vi "SubVI_SA_ReadMarker.vi"(8 "error in (no error)":errorcluster, 10 "AvgTimes":i32=1, 11 "VISA resource name":refnum<visa-resource-name>="TCPIP0::192.168.100.230::inst0::INSTR") -> (0 "error out":errorcluster, 1 "Marker Freq.":dbl, 3 "VISA resource name out":refnum<visa-resource-name>, 4 "Marker Power":dbl format="%.3f")   [LabVIEW 2023]
uses:
  Anritsu Signal Analyzer Series/Public/Data/Read Marker (Active Marker).vi
  Anritsu Signal Analyzer Series/Anritsu Signal Analyzer Series.lvlib
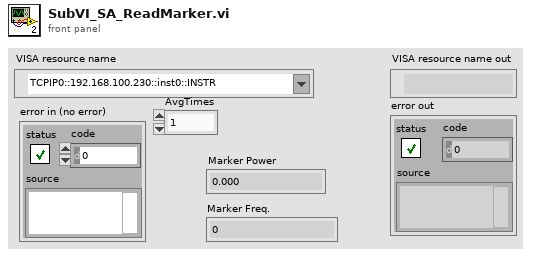
[diagram p1: front panel]
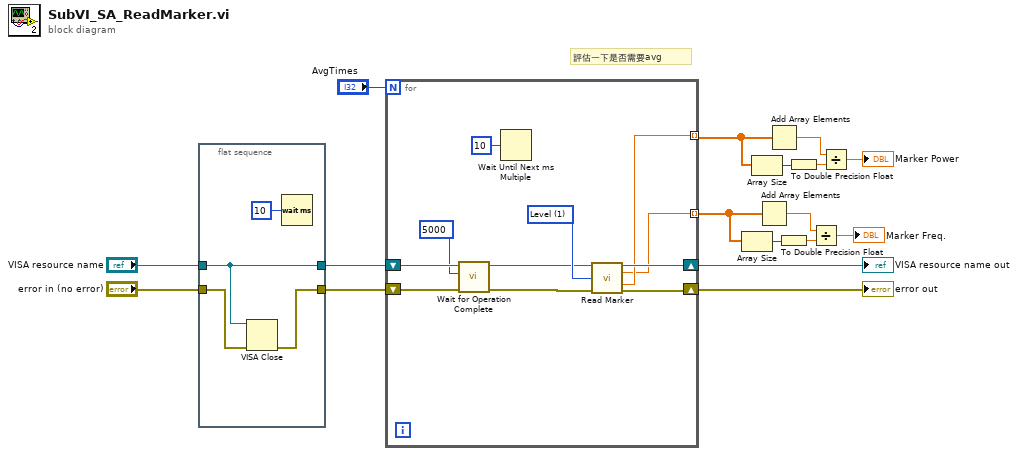
[diagram p0: block diagram]
diagram:
  # "評估一下是否需要avg"
  n1 = flat-sequence {
    tunnel: "error in (no error)" -> [w20]
    tunnel: [w19] -> w9
    tunnel: "VISA resource name" -> [w18]
    tunnel: [w18] -> w7
    frame #0 {
      n2 = VISA Close(VISA resource name=w18, error in (no error)=w20) -> (error out=w19:errorcluster)
      n3 = Wait (ms)(milliseconds to wait=u32 10) -> ()  [unwired: 1 out]
    }
  }
  n4 = for {
    N: "AvgTimes" -> [_]
    shift-right: [w27] -> w17
    shift-left: w7 -> [w29]
    shift-right: [w26] -> w16
    shift-left: w9 -> [w28]
    tunnel: [w25] -> w15 mode=indexing
    tunnel: [w23] -> w1 mode=indexing
    w32 = 1 items=["Frequency or Time", "Level", "Position"] ("Marker Type (0:Frequency or Time)")
    n5 = call "Wait for Operation Complete.vi"("error in (no error)"=w28, "Maximum Time (10000mSec)"=5000, "VISA resource name"=w29) -> ("error out"=w30:errorcluster, "VISA resource name out"=w31:refnum<visa-resource-name>)  [unwired: 7 in]
    n6 = Wait Until Next ms Multiple(millisecond multiple=u32 10) -> ()  [unwired: 1 out]
    n7 = call-poly "Read Marker.vi"("VISA resource name"=w31, "Marker Type (0:Frequency or Time)"=w32, "error in (no error)"=w30) -> ("VISA resource name out"=w27:refnum<visa-resource-name>, "Marker_X Response"=w23:dbl, "Marker_Y Response 2"=w25:dbl, "error out"=w26:errorcluster)  [unwired: 9 in]
  }
  "VISA resource name out" <- w17
  "error out" <- w16
  n8 = Array Size(array=w1) -> (size(s)=w4:i32)
  n9 = Array Size(array=w15) -> (size(s)=w13:i32)
  n10 = Add Array Elements(numeric array=w1) -> (sum=w3:dbl)
  n11 = Add Array Elements(numeric array=w15) -> (sum=w14:dbl)
  n12 = To Double Precision Float(number=w4) -> (double precision float=w5:dbl)
  n13 = To Double Precision Float(number=w13) -> (double precision float=w6:dbl)
  n14 = Divide(x=w3, y=w5) -> (x/y=→"Marker Freq.":dbl)
  n15 = Divide(x=w14, y=w6) -> (x/y=→"Marker Power":dbl)
